vi "RefreshSystemConfigurationUI.vi"(8 "error in (no error)":errorcluster, 11 "HardwareSetup_modle001:HardwareSetup_modle001":refnum<class "HardwareSetup_model001.lvclass">) -> (0 "error out":errorcluster, 3 "HardwareSetup_modle001:HardwareSetup_modle001":refnum<class "HardwareSetup_model001.lvclass">)   [LabVIEW 2019, in "HardwareSetup_model001.lvlib" / "HardwareSetup_model001.lvclass"]
uses:
  HardwareSetup_model001.lvclass
  C:/Program Files (x86)/National Instruments/LabVIEW 2019/vi.lib/NI/Event Source Actor/Event Source/Event Source/Event Source.lvclass
  InstrumentCommunication.lvclass
  C:/Program Files (x86)/National Instruments/LabVIEW 2019/vi.lib/NI/Event Source Actor/Event Source/Event/Event.lvclass
  <vilib>/NI/Event Source Actor/Event Source/Event/Event.lvclass/Event.ctl
  HardwareSetup_model001.lvclass/HardwareSetup_model001.ctl
  SystemSetup/SystemSetup/SystemSetup.lvclass
  <vilib>/NI/Event Source Actor/Event Source/Event/Event.lvclass
  <vilib>/NI/Event Source Actor/Event Source/Event Source/Event Source.lvclass
  <vilib>/Utility/config.llb/NI_LVConfig.lvlib
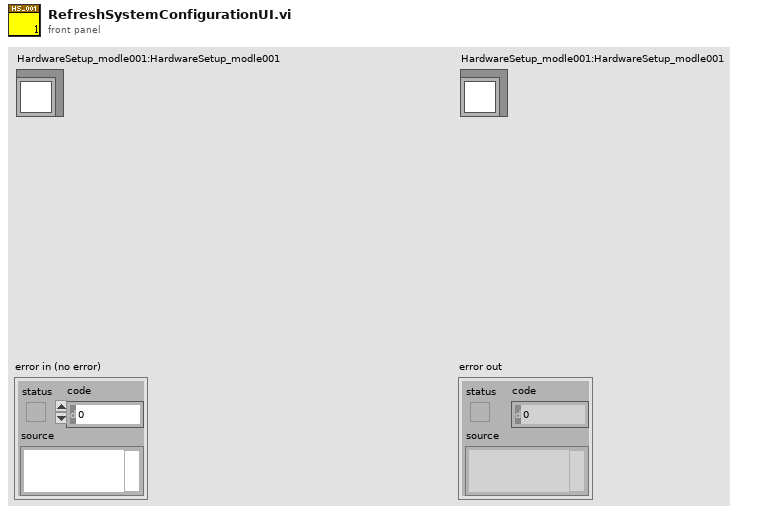
[diagram p1: front panel]
types:
  T1 = typedef "HardwareSetup_model001.lvlib/LIN.ctl" = cluster{"LIN 1":cluster{"Instrument model":string, "Port":string, "Baud rate":i32, "ID":i32, "Terminal":bool}, "LIN 2":cluster{"Instrument model":string, "Port":string, "Baud rate":i32, "ID":i32, "Terminal":bool}, "LIN 3":cluster{"Instrument model":string, "Port":string, "Baud rate":i32, "ID":i32, "Terminal":bool}, "LIN 4":cluster{"Instrument model":string, "Port":string, "Baud rate":i32, "ID":i32, "Terminal":bool}}
  T2 = typedef "HardwareSetup_model001.lvlib/Digital IO.ctl" = cluster{"Digital IO 1":cluster{"SerialPort":string, "Baud rate":i32, "Address":string, "ID":i32, "Port":i32, "Instrument model":string}, "Digital IO 2":cluster{"SerialPort":string, "Baud rate":i32, "Address":string, "ID":i32, "Port":i32, "Instrument model":string}, "Digital IO 3":cluster{"SerialPort":string, "Baud rate":i32, "Address":string, "ID":i32, "Port":i32, "Instrument model":string}, "Digital IO 4":cluster{"SerialPort":string, "Baud rate":i32, "Address":string, "ID":i32, "Port":i32, "Instrument model":string}}
  T3 = typedef "HardwareSetup_model001.lvlib/DMM.ctl" = cluster{"DMM 1":cluster{"SerialPort":string, "Baud rate":i32, "Address":string, "ID":i32, "Port":i32, "Instrument model":string}, "DMM 2":cluster{"SerialPort":string, "Baud rate":i32, "Address":string, "ID":i32, "Port":i32, "Instrument model":string}, "DMM 3":cluster{"SerialPort":string, "Baud rate":i32, "Address":string, "ID":i32, "Port":i32, "Instrument model":string}, "DMM 4":cluster{"SerialPort":string, "Baud rate":i32, "Address":string, "ID":i32, "Port":i32, "Instrument model":string}}
  T4 = typedef "HardwareSetup_model001.lvlib/Oscilloscope.ctl" = cluster{"Oscilloscope 1":cluster{"SerialPort":string, "Baud rate":i32, "Address":string, "ID":i32, "Port":i32, "Instrument model":string}, "Oscilloscope 2":cluster{"SerialPort":string, "Baud rate":i32, "Address":string, "ID":i32, "Port":i32, "Instrument model":string}, "Oscilloscope 3":cluster{"SerialPort":string, "Baud rate":i32, "Address":string, "ID":i32, "Port":i32, "Instrument model":string}, "Oscilloscope 4":cluster{"SerialPort":string, "Baud rate":i32, "Address":string, "ID":i32, "Port":i32, "Instrument model":string}}
  T5 = typedef "HardwareSetup_model001.lvlib/PLC.ctl" = cluster{"PLC 1":cluster{"SerialPort":string, "Baud rate":i32, "Address":string, "ID":i32, "Port":i32, "Instrument model":string}}
  T6 = typedef "HardwareSetup_model001.lvlib/ElectronicLoad.ctl" = cluster{"ElectronicLoad 1":cluster{"SerialPort":string, "Baud rate":i32, "Address":string, "ID":i32, "Port":i32, "Instrument model":string}, "ElectronicLoad 2":cluster{"SerialPort":string, "Baud rate":i32, "Address":string, "ID":i32, "Port":i32, "Instrument model":string}, "ElectronicLoad 3":cluster{"SerialPort":string, "Baud rate":i32, "Address":string, "ID":i32, "Port":i32, "Instrument model":string}, "ElectronicLoad 4":cluster{"SerialPort":string, "Baud rate":i32, "Address":string, "ID":i32, "Port":i32, "Instrument model":string}}
  T7 = typedef "HardwareSetup_model001.lvlib/PowerSupply.ctl" = cluster{"PowerSupply 1":cluster{"SerialPort":string, "Baud rate":i32, "Address":string, "ID":i32, "Port":i32, "Instrument model":string}, "PowerSupply 2":cluster{"SerialPort":string, "Baud rate":i32, "Address":string, "ID":i32, "Port":i32, "Instrument model":string}, "PowerSupply 3":cluster{"SerialPort":string, "Baud rate":i32, "Address":string, "ID":i32, "Port":i32, "Instrument model":string}, "PowerSupply 4":cluster{"SerialPort":string, "Baud rate":i32, "Address":string, "ID":i32, "Port":i32, "Instrument model":string}}
  T8 = typedef "HardwareSetup_model001.lvlib/CAN.ctl" = cluster{"CAN 1":cluster{"Instrument model":string, "Port":string, "Baud rate":i32, "ID":i32, "Terminal":bool}, "CAN 2":cluster{"Instrument model":string, "Port":string, "Baud rate":i32, "ID":i32, "Terminal":bool}, "CAN 3":cluster{"Instrument model":string, "Port":string, "Baud rate":i32, "ID":i32, "Terminal":bool}, "CAN 4":cluster{"Instrument model":string, "Port":string, "Baud rate":i32, "ID":i32, "Terminal":bool}}
  T9 = typedef "HardwareSetup_model001.lvlib/Programming.ctl" = cluster{"Programming 1":cluster{"Test Image":string, "Address":string, "Port":i32, "Instrument model":string, "Final Image":string}, "Programming 2":cluster{"Test Image":string, "Address":string, "Port":i32, "Instrument model":string, "Final Image":string}}
  T10 = typedef "HardwareSetup_model001.lvlib/Scanner.ctl" = cluster{"Scanner 1":cluster{"SerialPort":string, "Baud rate":i32, "Address":string, "ID":i32, "Port":i32, "Instrument model":string}, "Scanner 2":cluster{"SerialPort":string, "Baud rate":i32, "Address":string, "ID":i32, "Port":i32, "Instrument model":string}, "Scanner 3":cluster{"SerialPort":string, "Baud rate":i32, "Address":string, "ID":i32, "Port":i32, "Instrument model":string}, "Scanner 4":cluster{"SerialPort":string, "Baud rate":i32, "Address":string, "ID":i32, "Port":i32, "Instrument model":string}}
  T11 = cluster{"LIN":T1, "Digital IO":T2, "DMM":T3, "Oscilloscope":T4, "PLC":T5, "ElectronicLoad":T6, "PowerSupply":T7, "CAN":T8, "Programming":T9, "Scanner":T10}
  T12 = typedef "NI_LVConfig.lvlib/Config Data RefNum.ctl" = refnum<k1>
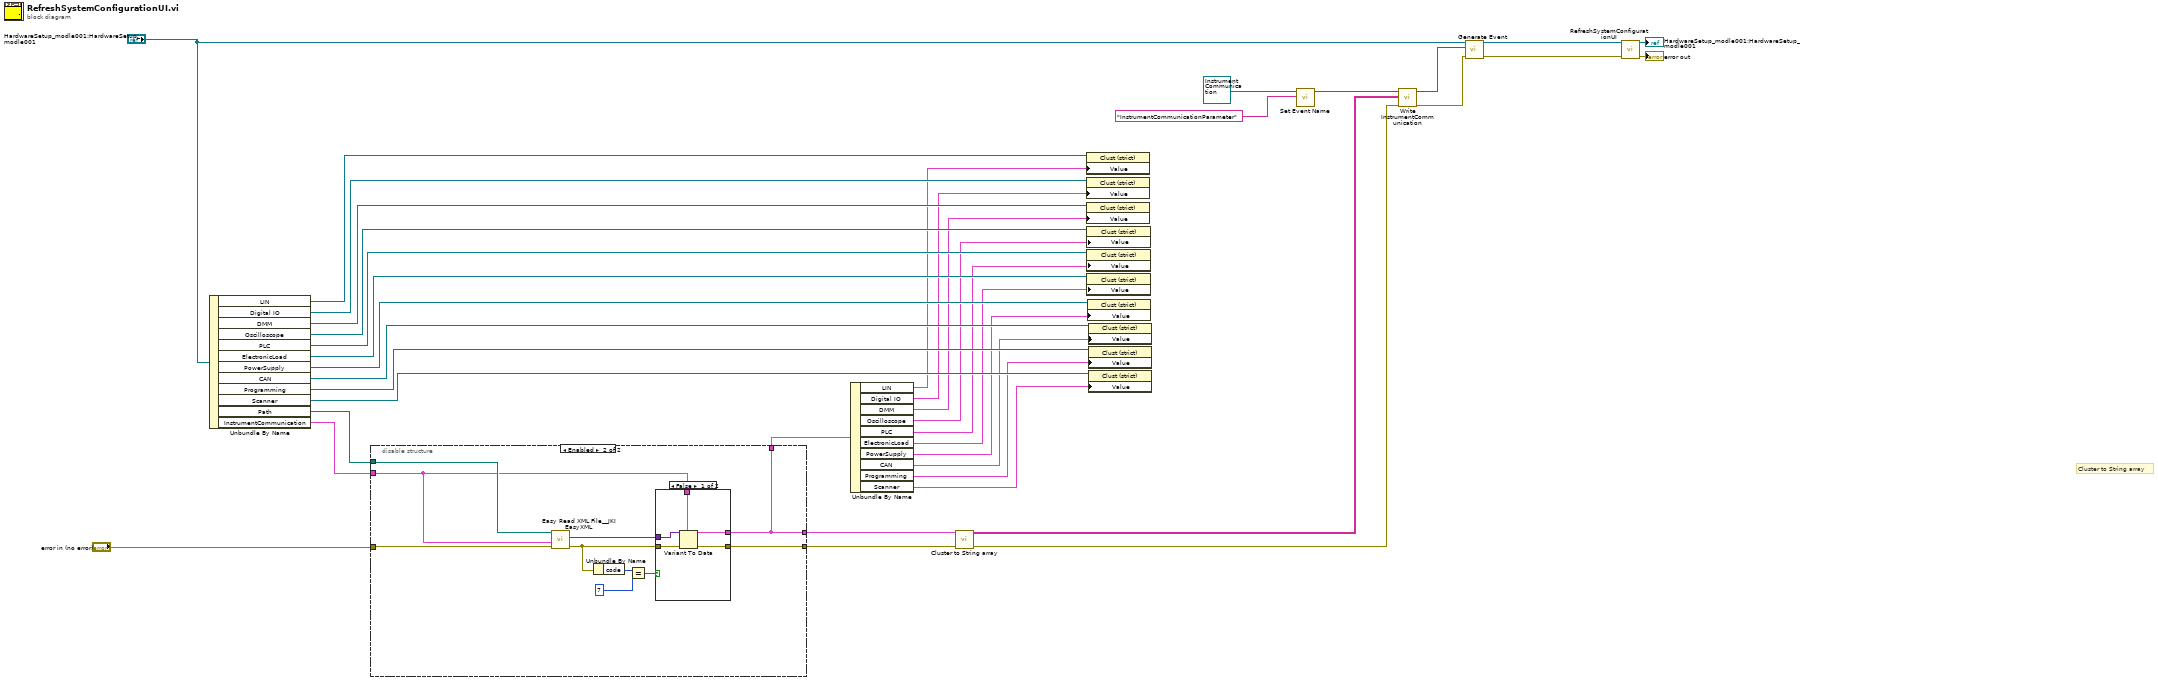
[diagram p0: block diagram]
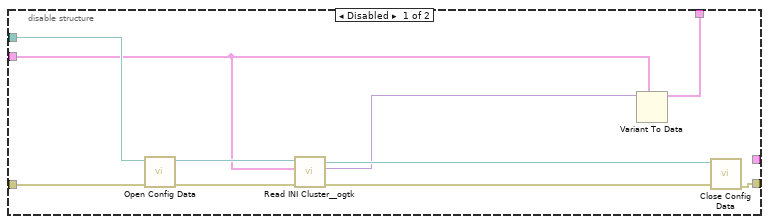
[diagram p2: hidden frame]
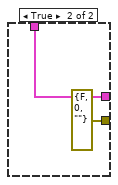
[diagram p3: hidden frame]
diagram:
  # "Cluster to String array"
  n1 = Unbundle By Name("HardwareSetup_modle001:HardwareSetup_modle001") -> ("LIN"=w27:refnum<vi>, "Digital IO"=w26:refnum<vi>, "DMM"=w25:refnum<vi>, "Oscilloscope"=w24:refnum<vi>, "PLC"=w23:refnum<vi>, "ElectronicLoad"=w22:refnum<vi>, "PowerSupply"=w21:refnum<vi>, "CAN"=w20:refnum<vi>, "Programming"=w19:refnum<vi>, "Scanner"=w18:refnum<vi>, "Path"=w32:path, "InstrumentCommunication"=w31:T11)
  n2 = disable-structure shown="Enabled" {
    disable-tunnel: w32 -> [w42 w56]
    disable-tunnel: "error in (no error)" -> [w41 w57]
    disable-tunnel: [w40 w53] -> w29
    disable-tunnel: [w39 w48] -> w28
    disable-tunnel: w31 -> [w38 w54]
    disable-tunnel: [_ w48] -> w2
    frame Disabled {
      n3 = call <vilib>:"Open Config Data.vi"("error in (no error)"=w41, "configuration file path"=w42) -> ("error out"=w46:errorcluster, "refnum"=w47:T12)  [unwired: 7 in, 1 out]
      n4 = call <userlib>:"Read INI Cluster__ogtk.vi"("error in (no error)"=w46, "INI Fomatted Cluster Type"=w38, "refnum"=w47) -> ("error out"=w44:errorcluster, "INI Fomatted Cluster"=w43:variant, "dup refnum"=w45:T12)  [unwired: 4 in, 2 out]
      n5 = Variant To Data(type=w38, Variant=w43) -> (data=w39:T11)  [unwired: 1 in, 1 out]
      n6 = call <vilib>:"Close Config Data.vi"("error in (no error)"=w44, "refnum"=w45) -> ("error out"=w40:errorcluster)  [unwired: 8 in, 1 out]
    }
    frame Enabled {
      n7 = call <vilib>:"Easy Read XML File__JKI EasyXML.vi"("error in (no error)"=w57, "LabVIEW Data (Type)"=w54, "XML File Path"=w56) -> ("error out"=w49:errorcluster, "LabVIEW Data"=w55:variant)  [unwired: 6 in, 1 out]
      n8 = Unbundle By Name(w49) -> ("code"=w52:i32)
      n9 = Equal?(x=w52, y=7) -> (x = y?=w50:bool)
      n10 = case shown="False" w50 {
        tunnel: w55 -> [w62 _]
        tunnel: w54 -> [w61 w64]
        tunnel: [w60 w64] -> w48
        tunnel: [w59 errorcluster {"status"=FALSE, "code"=0, "source"=""} ("error out")] -> w53
        tunnel: w49 -> [w58 _]
        frame False {
          n11 = Variant To Data(error in=w58, type=w61, Variant=w62) -> (data=w60:T11, error out=w59:errorcluster)
        }
        frame True {
        }
      }
    }
  }
  n12 = Unbundle By Name(w28) -> ("LIN"=w3:T1, "Digital IO"=w6:T2, "DMM"=w12:T3, "Oscilloscope"=w11:T4, "PLC"=w10:T5, "ElectronicLoad"=w9:T6, "PowerSupply"=w8:T7, "CAN"=w5:T8, "Programming"=w4:T9, "Scanner"=w7:T10)
  n13 = call "Cluster to String array.vi"("input cluster"=w2) -> ("appended array"=w1:string[][])  [unwired: 10 in]
  n14 = property class="Clust (strict)"(reference=w27, "Value"=w3) -> ()  [unwired: 1 in, 2 out]
  n15 = property class="Clust (strict)"(reference=w26, "Value"=w6) -> ()  [unwired: 1 in, 2 out]
  n16 = property class="Clust (strict)"(reference=w25, "Value"=w12) -> ()  [unwired: 1 in, 2 out]
  n17 = property class="Clust (strict)"(reference=w24, "Value"=w11) -> ()  [unwired: 1 in, 2 out]
  n18 = property class="Clust (strict)"(reference=w23, "Value"=w10) -> ()  [unwired: 1 in, 2 out]
  n19 = property class="Clust (strict)"(reference=w22, "Value"=w9) -> ()  [unwired: 1 in, 2 out]
  n20 = property class="Clust (strict)"(reference=w21, "Value"=w8) -> ()  [unwired: 1 in, 2 out]
  n21 = property class="Clust (strict)"(reference=w20, "Value"=w5) -> ()  [unwired: 1 in, 2 out]
  n22 = property class="Clust (strict)"(reference=w19, "Value"=w4) -> ()  [unwired: 1 in, 2 out]
  n23 = property class="Clust (strict)"(reference=w18, "Value"=w7) -> ()  [unwired: 1 in, 2 out]
  n24 = call <vilib>:"Set Event Name.vi"("Name (Generic)"="InstrumentCommunicationParameter", "Event In"=refnum<class "InstrumentCommunication.lvclass"> refnum ("HardwareSetup_bench001.lvlib:InstrumentCommunication.lvclass")) -> ("Event Out"=w15:refnum<class "InstrumentCommunication.lvclass">)  [unwired: 9 in]
  n25 = call-dynamic "Write InstrumentCommunication.vi"("error in (no error)"=w29, "InstrumentCommunication"=w1, "InstrumentCommunication in"=w15) -> ("error out"=w13:errorcluster, "InstrumentCommunication out"=w14:refnum<class "InstrumentCommunication.lvclass">)  [unwired: 7 in]
  n26 = call <vilib>:"Generate Event.vi"("Error In"=w13, "Event"=w14, "Event Source In"="HardwareSetup_modle001:HardwareSetup_modle001") -> ("Error Out"=w33:errorcluster, "Event Source Out"=w34:refnum<class "HardwareSetup_model001.lvclass">)  [unwired: 7 in]
  n27 = call-parent "RefreshSystemConfigurationUI.vi"("error in (no error)"=w33, "SystemSetup in"=w34) -> ("error out"=→"error out":errorcluster, "SystemSetup out"=→"HardwareSetup_modle001:HardwareSetup_modle001":refnum<class "HardwareSetup_model001.lvclass">)  [unwired: 8 in]
